vi "ble_discover_handle_tablePROVA.vi"() -> (2 "Handle table":string[][](array[string]))   [LabVIEW 2016]
panel:
  out "element":u8
  out "Array":string[][](array[string])
  out "initialized array":string[](array[string])
  out "HEX string OUT":string
  in  "service_info":u8[][](array[numeric])=[[0, 1, 0, 5, 0, 2, 1, 24], [0, 20, 0, 28, 0, 2, 0, 24], [0, 40, 0, 43, 0, 2, 255, 0], [0, 44, 0, 255, 255, 2, 223, 0]] format="%02d"
  in  "characteristics_info":u8[][](array[numeric]) format="%02x"
  # "4 - 8 - 3 - 3"
  # "3 - 7 - 4 - 4"
  # "service info"
  # "handle table"
  # "da 1 a 3"
  # "da 1 a 5"
  # "5 - 9 - 4"
  # "4 - 8 - 4 -"
  # "da 20 a 26"
  # "da 20 a 28"
  # "da 40 a 43"
  # "da 40 a 43"
  # "5-9-5-"
  # "da 44 a Inf"
  # "da 44 a 47"
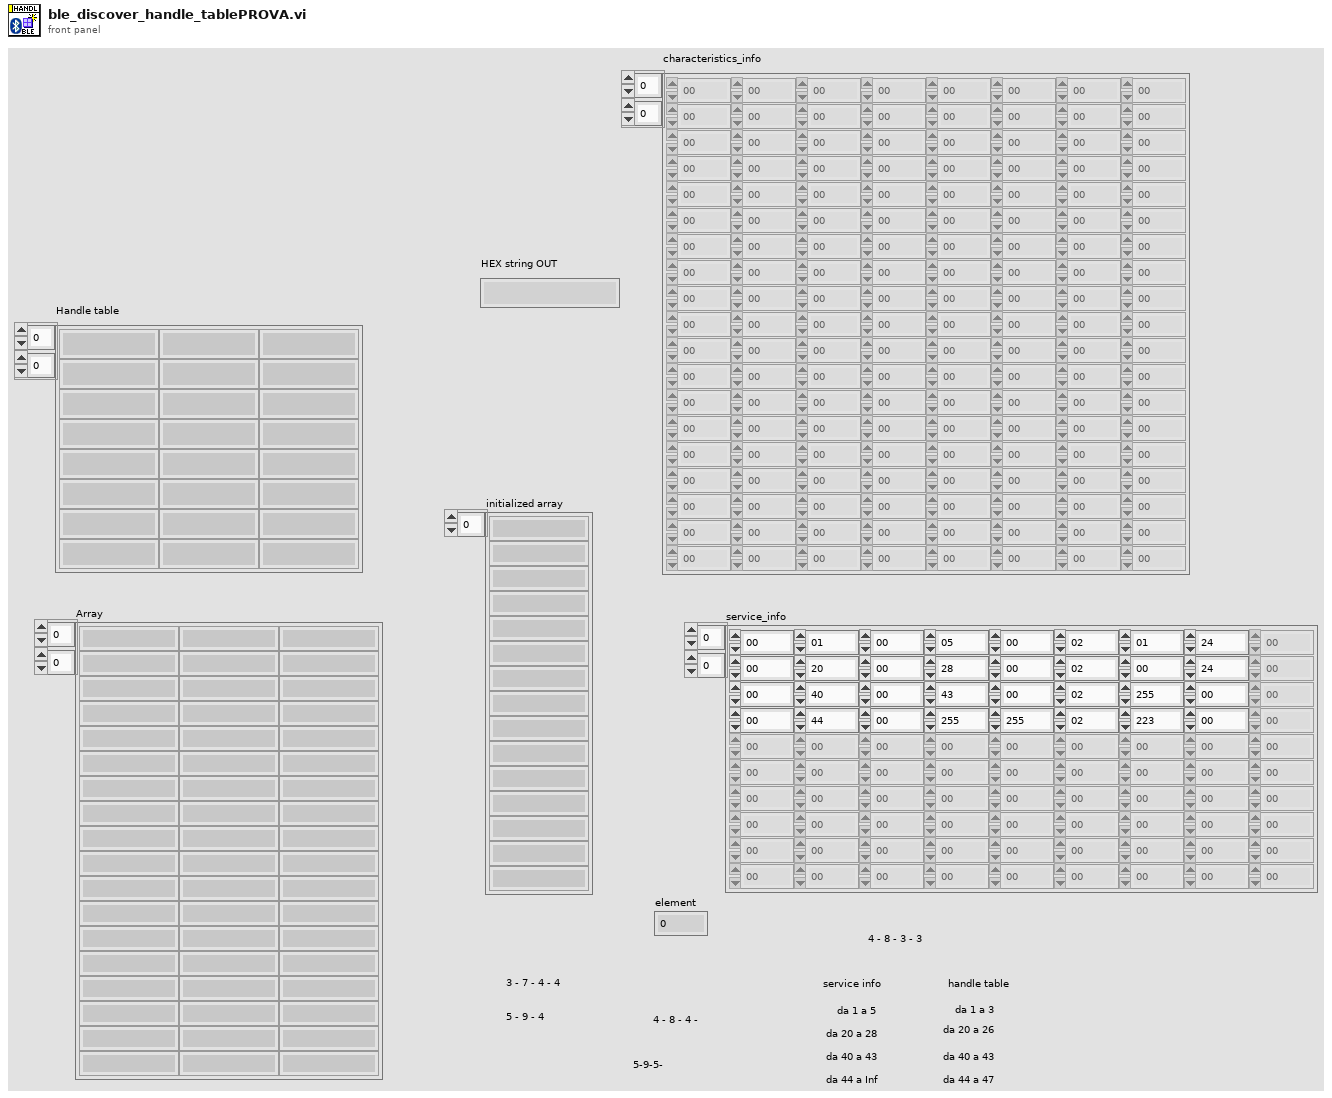
[diagram p1: front panel]
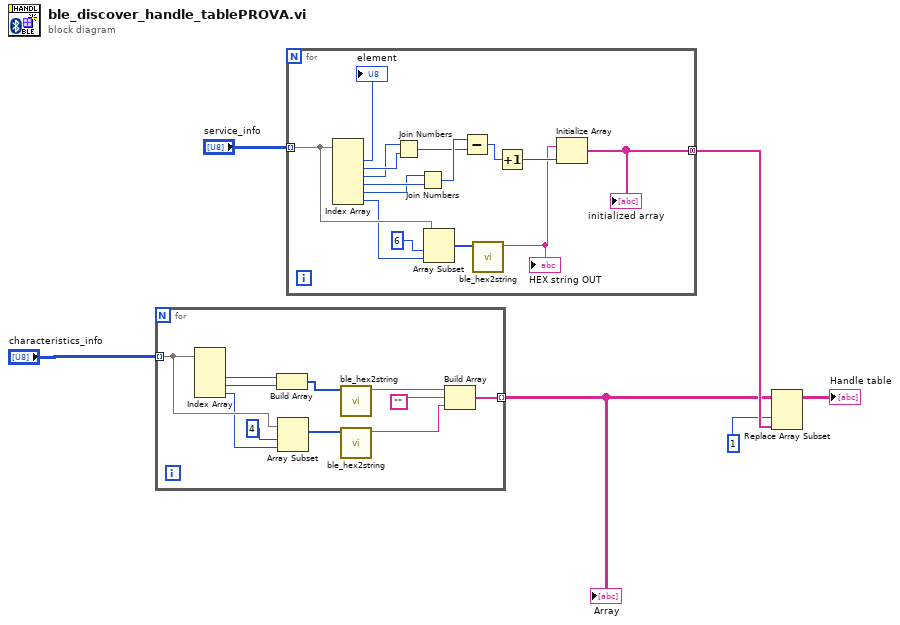
[diagram p0: block diagram]
diagram:
  n1 = for {
    tunnel: "characteristics_info" -> [w17] mode=indexing
    tunnel: [w15] -> w5 mode=indexing
    n2 = Index Array(array=w17) -> (element #2=w12:u8, element #3=w13:u8, element #4=w14:u8)  [unwired: 4 in, 1 out]
    n3 = Build Array(w12, w13) -> (w8:u8[])
    n4 = Array Subset(array=w17, index=4, length=w14) -> (w9:u8[])
    n5 = call <vilib>:"ble_hex2string.vi"("Byte Array IN (index0 LS byte)"=w8) -> ("HEX string OUT"=w7:string)  [unwired: 10 in]
    n6 = call <vilib>:"ble_hex2string.vi"("Byte Array IN (index0 LS byte)"=w9) -> ("HEX string OUT"=w10:string)  [unwired: 10 in]
    n7 = Build Array(w7, "", w10) -> (w15:string[])
  }
  "Array" <- w5
  n8 = for {
    tunnel: "service_info" -> [w31] mode=indexing
    tunnel: [w27] -> w6 mode=concatenating
    n9 = Index Array(array=w31) -> (element #1=→"element":u8, element #2=w22:u8, element #3=w21:u8, element #4=w20:u8, element #5=w19:u8, element #6=w30:u8)  [unwired: 6 in]
    n10 = Join Numbers(hi=w21, lo=w22) -> ((hi.lo)=w25:u16)
    n11 = Join Numbers(hi=w19, lo=w20) -> ((hi.lo)=w26:u16)
    n12 = Array Subset(array=w31, index=6, length=w30) -> (w24:u8[])
    n13 = Subtract(x=w26, y=w25) -> (x-y=w32:u16)
    n14 = call <vilib>:"ble_hex2string.vi"("Byte Array IN (index0 LS byte)"=w24) -> ("HEX string OUT"=w23:string)  [unwired: 10 in]
    "HEX string OUT" <- w23
    n15 = Increment(x=w32) -> (x+1=w28:u16)
    n16 = Initialize Array(w23, w28) -> (w27:string[])
    "initialized array" <- w27
  }
  n17 = Replace Array Subset(array=w5, new element=w6, index (col)=1 ("disabled index (col)")) -> (→"Handle table":string[][])  [unwired: 1 in]
